vi "XNET String To IO Name (ECU).vi"(3 "string":string) -> (0 "XNET ECU":refnum<k21>)   [LabVIEW 2018]
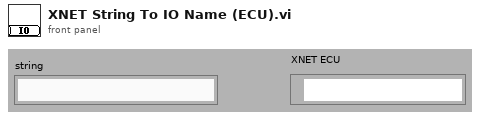
[diagram p1: front panel]
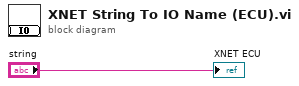
[diagram p0: block diagram]
diagram:
  "XNET ECU" <- "string"
